vi "IPS Reply to PGSQL.vi"(8 "error in (no error)":errorcluster, 10 "Response":T1, 11 "Instrument.VRM in":refnum<class "Instrument.OxfordVRM.lvclass">) -> (0 "error out":errorcluster, 3 "Instrument.VRM out":refnum<class "Instrument.OxfordVRM.lvclass">)   [LabVIEW 2016, in "Instrument.OxfordVRM.lvclass"]
uses:
  Instrument.OxfordVRM.lvclass
  <instrlib>/Mercury iXX/Public/Controls/Response String.ctl
  C:/Program Files (x86)/National Instruments/LabVIEW 2016/user.lib/LevyLab/Levylab Instruments/SMOs/Instrument/Instrument.lvclass
  <userlib>/LevyLab/Levylab Instruments/SMOs/Instrument/Instrument.lvclass
  <instrlib>/Mercury iXX/Mercury iXX.lvlib
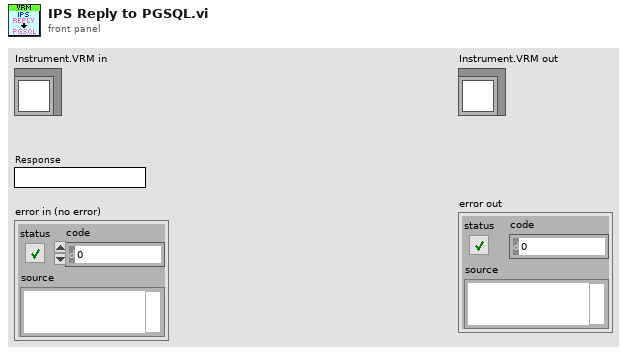
[diagram p1: front panel]
types:
  T1 = typedef "Mercury iXX.lvlib/Response String.ctl" = string
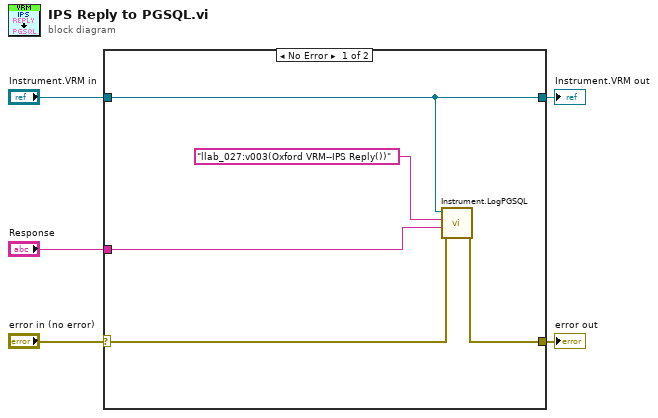
[diagram p0: block diagram]
diagram:
  n1 = case shown="No Error" "error in (no error)" {
    selector: "error in (no error)" -> [w6 w11]
    tunnel: "Response" -> [w7 _]
    tunnel: [w8 w11] -> w4
    tunnel: "Instrument.VRM in" -> [w10 w12]
    tunnel: [w10 w12] -> w1
    frame No Error {
      n2 = call <userlib>:"Instrument.LogPGSQL.vi"("error in (no error)"=w6, "Data"=w7, "Path"="llab_027:v003(Oxford VRM--IPS Reply())" ("variable"), "Instrument"=w10) -> ("error out"=w8:errorcluster)  [unwired: 6 in, 1 out]
    }
    frame Error {
    }
  }
  "error out" <- w4
  "Instrument.VRM out" <- w1
